vi "gui_T2.vi"(10 "input_xyz":T1) -> ()   [LabVIEW 2018]
uses:
  <vilib>/Analysis/NI_AALBase.lvlib
panel:
  in  "MW_power_db":dbl=1.0 caption="Width" min=0.0 max=10000.0 format="%#.3f"
  in  "MW_frequency_GHZ":dbl=1.0 caption="Width" min=0.0 max=10000.0 format="%#.3f"
  in  "Measurement_mode":enum16{"T2", "Rabi"}(ring)=enum."Rabi"
  in  "recenter_period_s":u32=5
  in  "recenter":bool=TRUE
  in  "show_all":bool
  in  "hide_all":bool
  out "elapsed_time_HMS":string
  in  "initial parameters":dbl[](array[numeric])=[0.5, 0.0001, 2.0, 100.0]
  out "estimated_time_HMS":string
  in  "plot_pulses":bool
  in  "gates_calculation":enum16{"Software", "Hardware"}(ring)=enum."Hardware"
  out "pulses":u32[][](graph)
  out "detections":u32[](graph)
  out "std. dev.":dbl format="%.3f"
  out "mean":dbl format="%0.2f"
  in  "auto_normalize":bool
  in  "normalize":bool
  in  "normalization_value":dbl=1.0 caption="Normalization value:" min=1.0 step=1.0
  out "status":string
  in  "use_proposed_width":bool
  in  "calc_width":bool
  in  "start":bool caption="Start"
  in  "save_file":bool
  out "contrast":dbl caption="Contrast :" format="%#_3f"
  in  "show_photons":bool
  in  "show_flags":bool
  out "mse":cluster{"read_widths_us":dbl[], "mse":dbl[]}(graph)
  in  "use_proposed_correction":bool
  out "proposed_read_width_us":dbl
  out "proposed_correction_us":dbl
  out "histogram":cluster{"histogram":i32[], "q_photons":i32[]}(graph)
  out "file_name":string caption="File name :"
  in  "sampling_mode":enum16{"Normal", "Sweep"}(ring)=enum."Sweep"
  out "quality":bool
  out "mse":dbl caption="Mean Square Error" format="%#.2e"
  out "T1_us":dbl format="%#.3g"
  out "T1 curves":cluster{dbl[], "dark_time_us":dbl[]}[](graph)
  in  "correction_us":dbl=0.65 caption="Delay"
  out "stop_count_photon":u32(colorbox)=16776704 caption="Stop Count & photon"
  out "stop_count":u32(colorbox)=6618880 caption="Stop Count"
  out "start_count_photon":u32(colorbox)=14417925 caption="Start Count & photon"
  out "start_count":u32(colorbox)=255 caption="Start Count"
  out "photon":u32(colorbox)=16448250 caption="Photon"
  out "noPhoton":u32(colorbox) caption="No Photon"
  out "photons_chart":u32[][](graph)
  in  "load_file":bool
  in  "refit":bool
  in  "read_width_us":dbl=1.0 caption="Width" min=0.0 max=10000.0 format="%#.3f"
  in  "read_delay_us":dbl caption="Delay"
  out "min_step":dbl format="%#.3f"
  in  "q_samples":i32=50
  in  "dt_stop_us":dbl=10000.0
  in  "dt_start_us":dbl=0.2
  in  "stop":bool
  in  "repetitions":i32=10000 caption="Repetitions" min=1 step=1
  in  "pulse_width_us":dbl=5.0 caption="Pulse width"
  # "Dark time [us]"
  # "*"
  # "*"
  # "us"
  # "*read_width_us and correction_us have to be multiple of 10ns\n*** start and stop markers are inside the detection gate. [start, stop]"
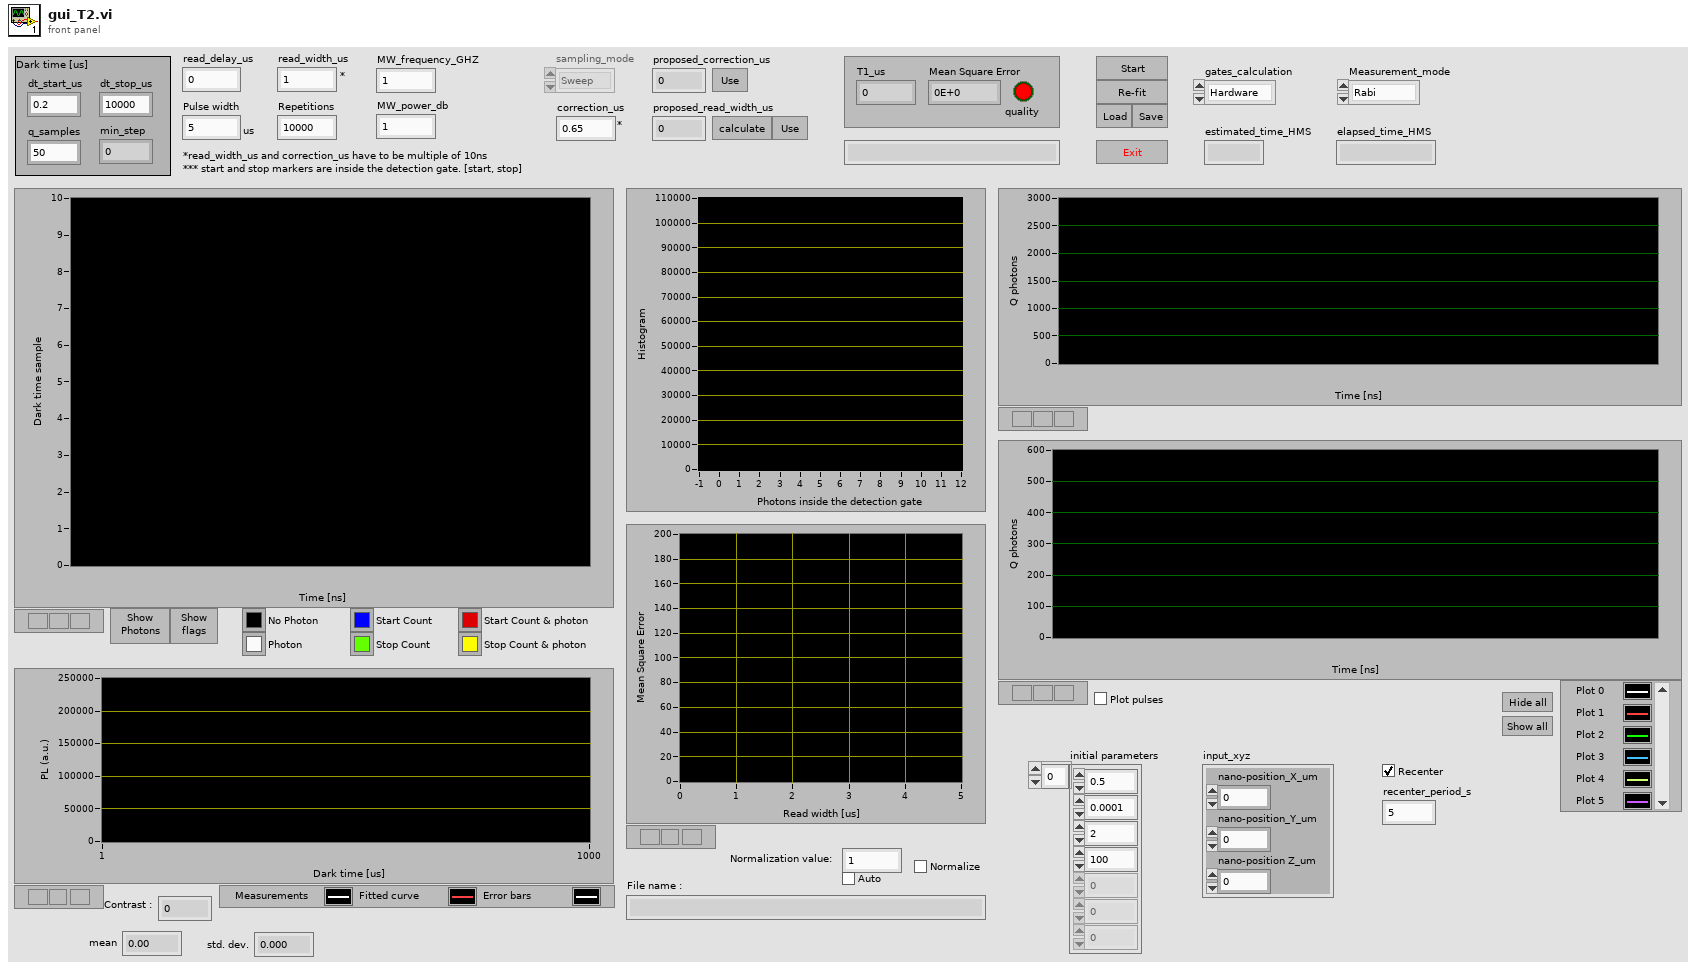
[diagram p1: front panel]
types:
  T1 = cluster{"nano-position_X_um":sgl, "nano-position_Y_um":sgl, "nano-position Z_um":sgl}
  T2 = cluster{"MW_power_db":dbl, "MW_frequency_GHZ":dbl}
  T3 = cluster{"MW_width_us":dbl[], "pulse_width_us":dbl, "read_delay_us":dbl, "read_width_us":dbl, "repetitions":i32, "sampling_mode":enum16{"Normal", "Sweep"}, "correction_us":dbl}
  T4 = cluster{"file_path":path, "file_name":string, "image":dbl[][][], "image_size_xy":cluster{"image_size_x_um":sgl, "image_size_y_um":sgl}, "pixel_dwell_time_ms":sgl, "Laser_power_mW":sgl, "pixel_size":dbl, "tile_ij":cluster{"tile_i":i32, "tile_j":i32}, "Objective":string, "ColorMarkers":cluster{dbl, u32}[], "timestamp":timestamp, "micro-position-xyz":cluster{"micro-position_x_mm":sgl, "micro-position_y_mm":sgl, "micro-position_z_mm":sgl}, "zero_xyz":cluster{"zero_x_mm":dbl, "zero_y_mm":dbl, "zero_z_mm":dbl}, "nano-position-xyz":cluster{"nano-position_x_V":sgl, "nano-position_y_V":sgl, "nano-position_z_V":sgl}, "Kxyz":cluster{"Kx_V/um":sgl, "Ky_V/um":sgl, "Kz_V/um":sgl}}
  T5 = cluster{"x_um":sgl[], "y_um":sgl[], "z_um":sgl[], "timetag":timestamp[]}
  T6 = cluster{"sampling_times":dbl[], "fitted_signal":dbl[]}
  T7 = cluster{"Ie":dbl, "Cm":dbl, "Tm":dbl, "C1":dbl, "T1":dbl, "mse":dbl}
  T8 = cluster{"dark_times_us":dbl[], "pulse_width_us":dbl, "read_delay_us":dbl, "read_width_us":dbl, "repetitions":i32, "sampling_mode":enum16{"Normal", "Sweep"}, "correction_us":dbl}
  T9 = cluster{"input_xyz":cluster{"nano-position_X_um":sgl, "nano-position_Y_um":sgl, "nano-position Z_um":sgl}, "recenter":bool, "recenter_s":u32}
  T10 = enum16{"standby", "doT1", "abort", "save", "re-fit", "load", "refresh", "use_proposed", "calcWidth"}
  T11 = cluster{"dark_times":dbl[], "fitted_signal":dbl[]}
  T12 = cluster{"dark_times_us":dbl[], "measured_signal":dbl[]}
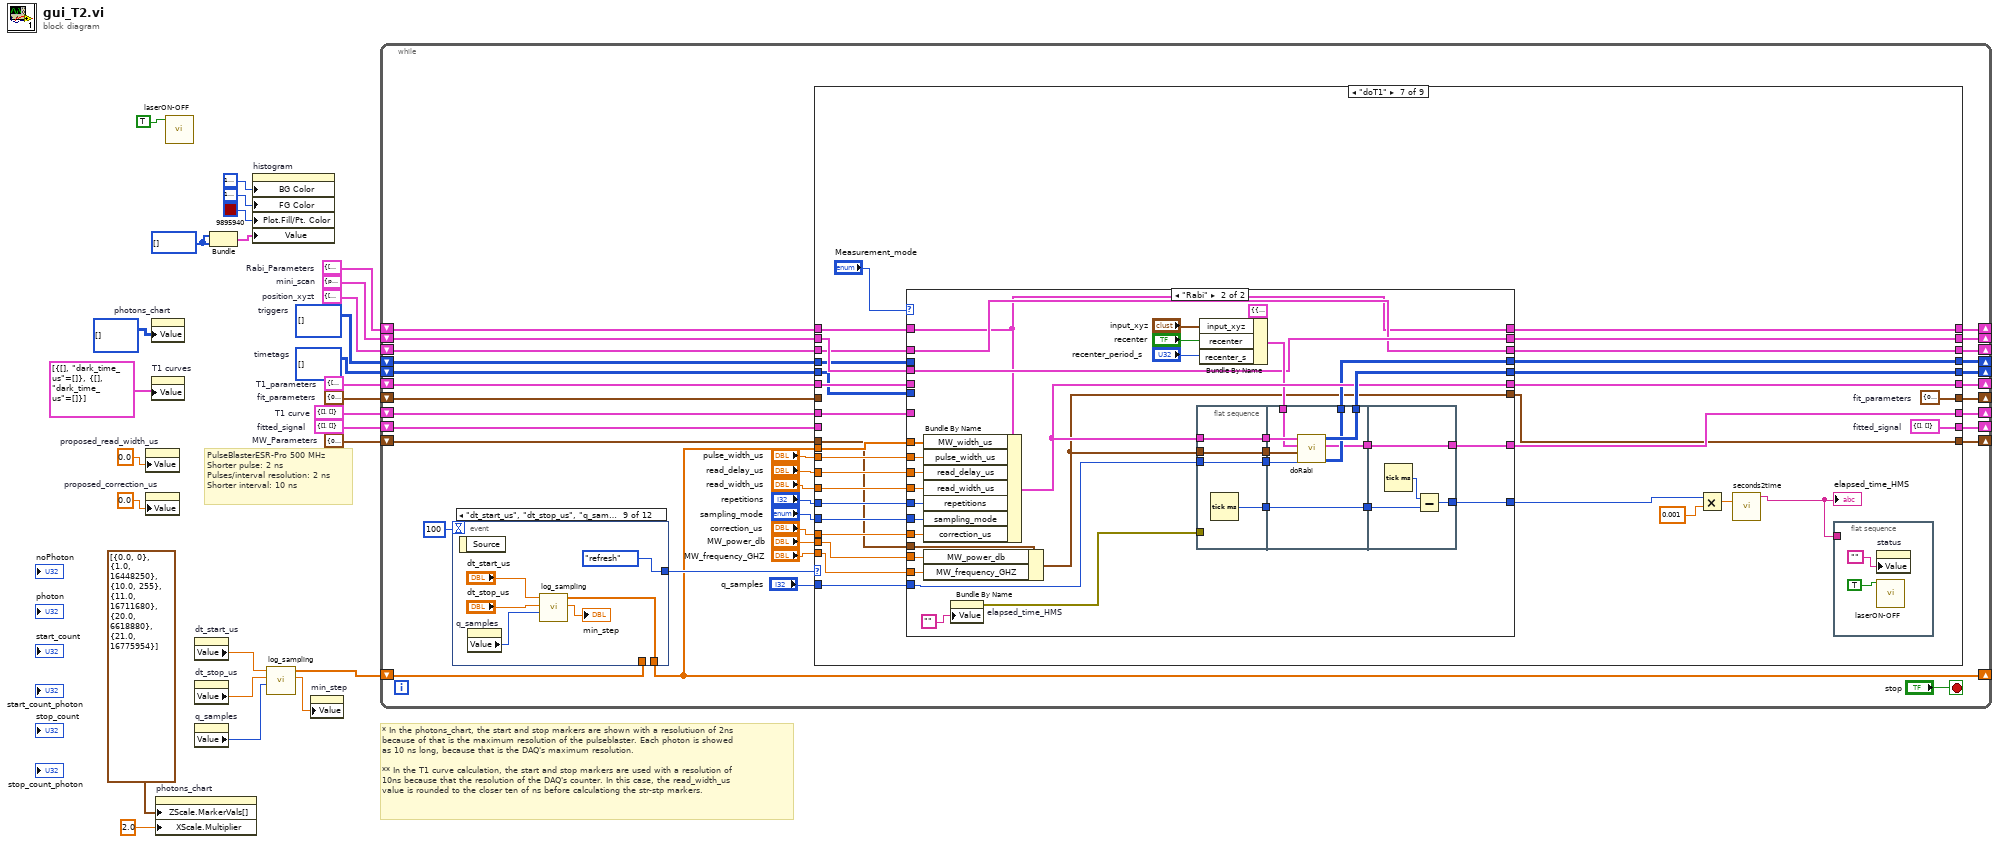
[diagram p0: block diagram]
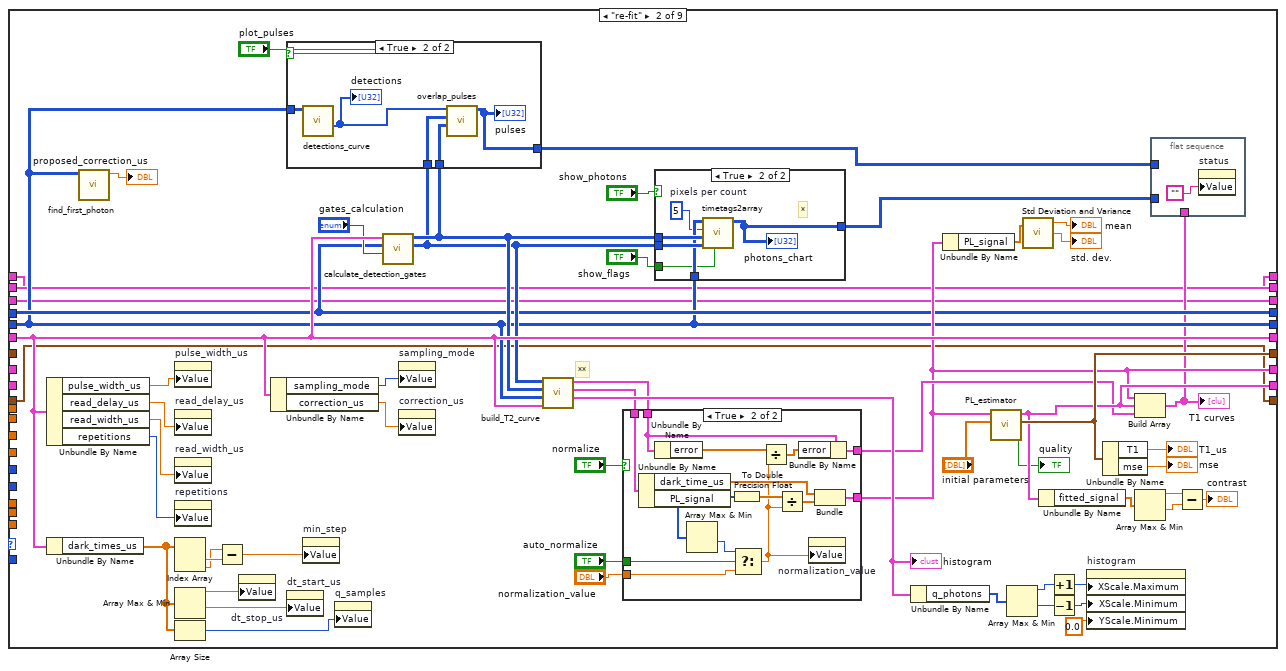
[diagram p3: hidden frame]
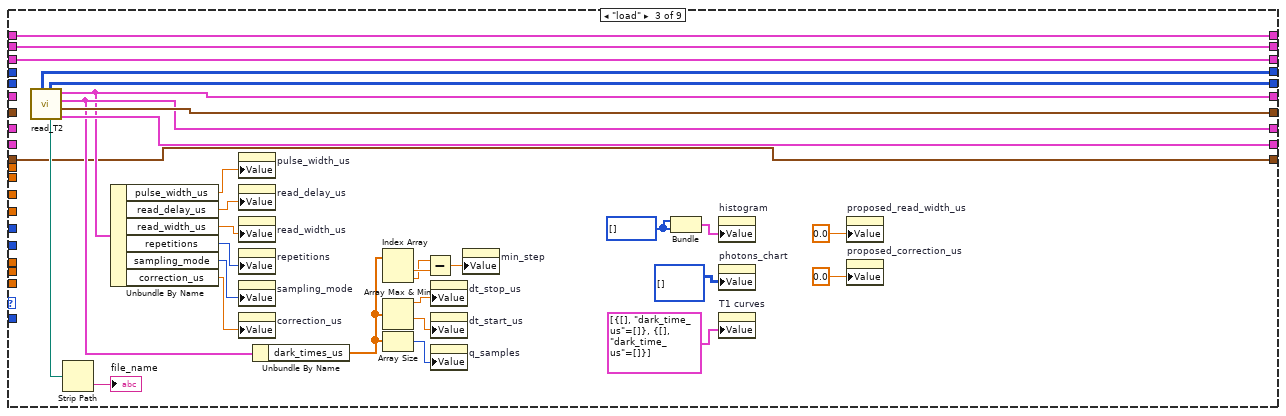
[diagram p7: hidden frame]
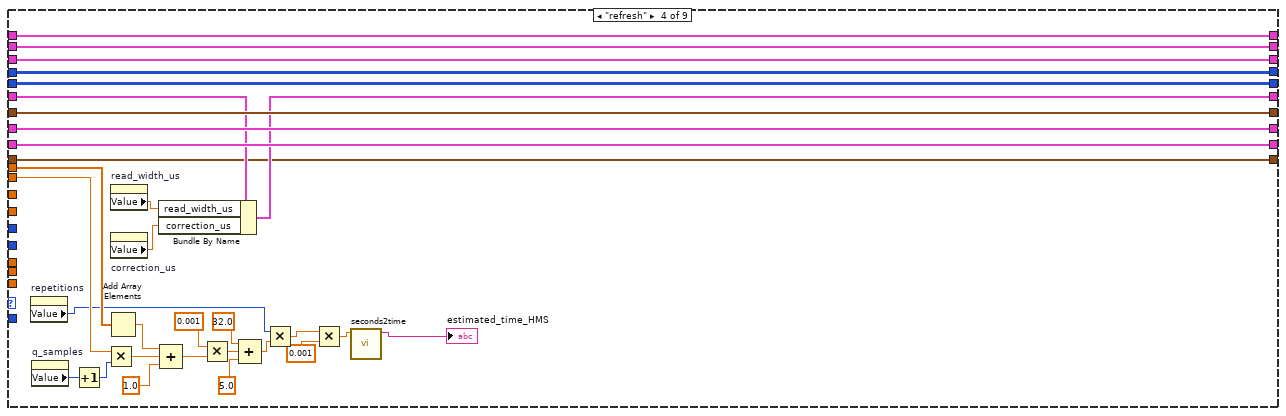
[diagram p8: hidden frame]
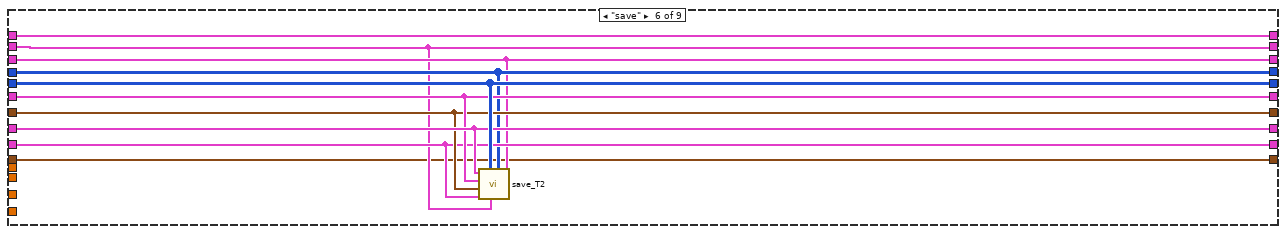
[diagram p10: hidden frame]
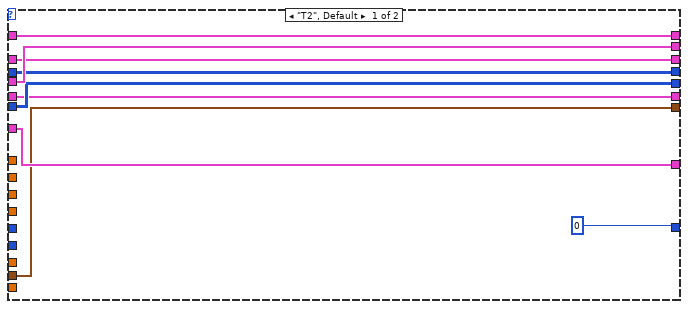
[diagram p11: hidden frame]
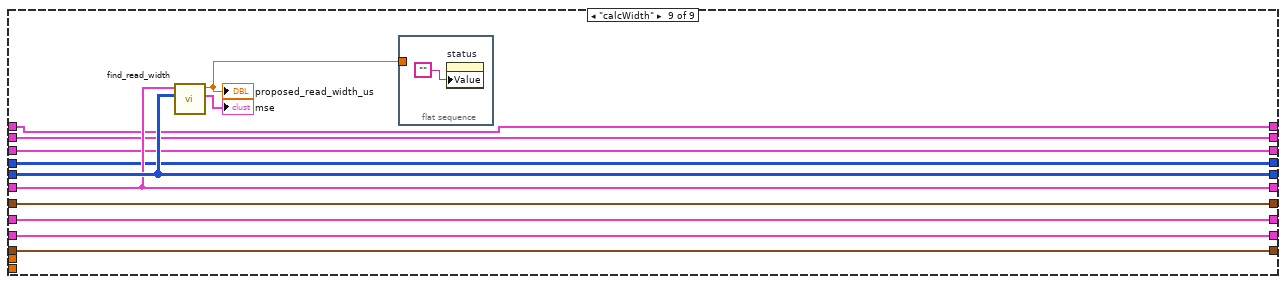
[diagram p13: hidden frame]
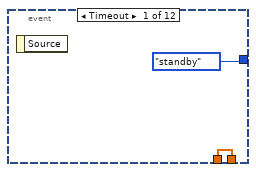
[diagram p14: hidden frame]
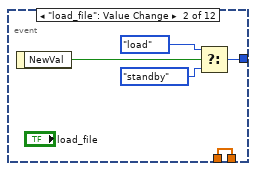
[diagram p15: hidden frame]
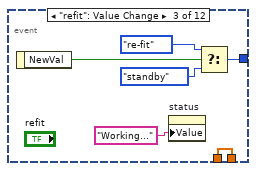
[diagram p16: hidden frame]
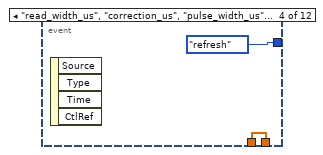
[diagram p17: hidden frame]
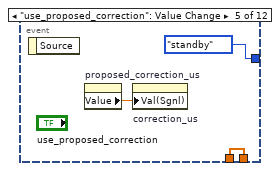
[diagram p18: hidden frame]
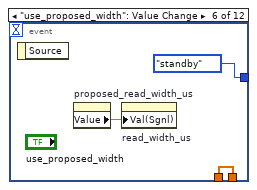
[diagram p19: hidden frame]
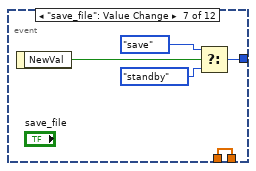
[diagram p20: hidden frame]
diagram:
  w1 = T2 {"MW_power_db"=0.0, "MW_frequency_GHZ"=0.0}  # MW_Parameters
  w2 = T3 {"MW_width_us"=[], "pulse_width_us"=0.0, "read_delay_us"=0.0, "read_width_us"=0.0, "repetitions"=0, "sampling_mode"=enum."Normal", "correction_us"=0.0}  # Rabi_Parameters
  w3 = T4 {"file_path"=path "", "file_name"="", "image"=[], "image_size_xy"={"image_size_x_um"=0.0, "image_size_y_um"=0.0}, "pixel_dwell_time_ms"=0.0, "Laser_power_mW"=0.0, "pixel_size"=0.0, "tile_ij"={"tile_i"=0, "tile_j"=0}, "Objective"="", "ColorMarkers"=[], "timestamp"=timestamp(0 s since 1904-01-01), "micro-position-xyz"={"micro-position_x_mm"=0.0, "micro-position_y_mm"=0.0, "micro-position_z_mm"=0.0}, "zero_xyz"={"zero_x_mm"=0.0, "zero_y_mm"=0.0, "zero_z_mm"=0.0}, "nano-position-xyz"={"nano-position_x_V"=0.0, "nano-position_y_V"=0.0, "nano-position_z_V"=0.0}, "Kxyz"={"Kx_V/um"=0.0, "Ky_V/um"=0.0, "Kz_V/um"=0.0}}  # mini_scan
  w4 = T5 {"x_um"=[], "y_um"=[], "z_um"=[], "timetag"=[]}  # position_xyzt
  w6 = u32[][] []  # triggers
  w24 = T6 {"sampling_times"=[], "fitted_signal"=[]}  # fitted_signal
  w7 = u32[][] []  # timetags
  w25 = cluster{dbl[], "dark_time_us":dbl[]} {[], "dark_time_us"=[]}  # T1 curve
  w26 = T7 {"Ie"=0.0, "Cm"=0.0, "Tm"=0.0, "C1"=0.0, "T1"=0.0, "mse"=0.0}  # fit_parameters
  w23 = T8 {"dark_times_us"=[], "pulse_width_us"=0.0, "read_delay_us"=0.0, "read_width_us"=0.0, "repetitions"=0, "sampling_mode"=enum."Normal", "correction_us"=0.0}  # T1_parameters
  w18 = i32[] []
  # "* In the photons_chart, the start and stop markers are shown with a resolutiuon of 2ns \nbecause of that is the maximum resolution of the pulseblaster. Each photon is showed\nas 10 ns long, because that is the DAQ's maximum resolution.\n\n** In the T1 curve calculation, the start and stop markers are used with a resolution of\n10ns because that the resolution of the DAQ's counter. In this case, the read_width_us\nvalue is rounded to the closer ten of ns before calculationg the str-stp markers."
  # "PulseBlasterESR-Pro 500 MHz \nShorter pulse: 2 ns\nPulses/interval resolution: 2 ns\nShorter interval: 10 ns"
  n1 = property on="proposed_read_width_us" class="DigNum (strict)"("Value"=0.0 ("proposed_read_width_us")) -> ()  [unwired: 2 in, 2 out]
  n2 = property on="proposed_correction_us" class="DigNum (strict)"("Value"=0.0 ("proposed_correction_us")) -> ()  [unwired: 2 in, 2 out]
  n3 = property on="photons_chart" class="IntGraph (strict)"("Value"=i32[][] []) -> ()  [unwired: 2 in, 2 out]
  n4 = property on="T1 curves" class="XYGraph (strict)"("Value"=cluster{dbl[], "dark_time_us":dbl[]}[] [{[], "dark_time_us"=[]}, {[], "dark_time_us"=[]}] ("T1 curves")) -> ()  [unwired: 2 in, 2 out]
  n5 = property on="photons_chart" class="IntGraph (strict)"("ZScale.MarkerVals[]"=cluster{dbl, u32}[] [{0.0, 0}, {1.0, 16448250}, {10.0, 255}, {11.0, 16711680}, {20.0, 6618880}, {21.0, 16775954}] ("Z Scale.Marker Values[]"), "XScale.Multiplier"=2.0 ("X Scale.Offset and Multiplier:Multiplier")) -> ()  [unwired: 2 in, 2 out]
  n6 = call "laserON-OFF.vi"("ON-OFF"=TRUE) -> ()  [unwired: 11 in]
  n7 = property on="dt_start_us" class="DigNum (strict)"() -> ("Value"=w10:dbl)  [unwired: 2 in, 2 out]
  n8 = property on="dt_stop_us" class="DigNum (strict)"() -> ("Value"=w11:dbl)  [unwired: 2 in, 2 out]
  n9 = property on="q_samples" class="DigNum (strict)"() -> ("Value"=w12:i32)  [unwired: 2 in, 2 out]
  n10 = Bundle(w18, w18) -> (w17:cluster{i32[], i32[]})  [unwired: 1 in]
  n11 = property on="histogram" class="XYGraph (strict)"("BG Color"=u32 16777222 ("Plot Area:Colors:FG Color"), "FG Color"=u32 16777228 ("Plot Area:Colors:FG Color"), "Plot.Fill/Pt. Color"=u32 9895940 ("Plot Area:Colors:FG Color"), "Value"=w17) -> ()  [unwired: 2 in, 2 out]
  n12 = call "log_sampling.vi"("q_samples"=w12, "stop_us"=w11, "start_us"=w10) -> ("min_step_us"=w13:dbl, "sampling_times_us"=w9:dbl[])  [unwired: 7 in]
  n13 = property on="min_step" class="DigNum (strict)"("Value"=w13) -> ()  [unwired: 2 in, 2 out]
  n14 = while {
    shift-right: [w51] -> _
    shift-left: w23 -> [w58]
    shift-right: [w50] -> _
    shift-left: w26 -> [w57]
    shift-right: [w49] -> _
    shift-left: w25 -> [w56]
    shift-right: [w55] -> _
    shift-left: w24 -> [w54]
    shift-right: [w52] -> _
    shift-left: w7 -> [w53]
    shift-right: [w41] -> _
    shift-left: w9 -> [w42]
    shift-right: [w40] -> _
    shift-left: w6 -> [w39]
    shift-right: [w38] -> _
    shift-left: w4 -> [w37]
    shift-right: [w35] -> _
    shift-left: w3 -> [w36]
    shift-right: [w33] -> _
    shift-left: w2 -> [w34]
    shift-right: [w29] -> _
    shift-left: w1 -> [w32]
    stop <- "stop" stop-if-true
    n15 = event shown="[8] \"dt_start_us\", \"dt_stop_us\", \"q_samples\": Value Change" {
      selector: _ -> [_ _ _ _ _ _ _ _ _ _ _ _]
      dyn-events: _ -> [_ _ _ _ _ _ _ _ _ _ _ _]
      timeout: 100 -> [_ _ _ _ _ _ _ _ _ _ _ _]
      tunnel: [T10."standby" w360 w366 T10."refresh" T10."standby" T10."standby" w379 w386 T10."refresh" w398 T10."standby" T10."standby"] -> w59
      tunnel: w42 -> [w355 w357 w363 w368 w370 w373 w376 w381 _ w394 w401 w407]
      tunnel: [w355 w357 w363 w368 w370 w373 w376 w381 w388 w394 w401 w407] -> w41
      event Timeout {
        n16 = event-data() -> ()  [unwired: 1 in, 1 out]
      }
      event "load_file": Value Change {
        n17 = event-data() -> ("NewVal"=w361:bool)  [unwired: 1 in]
        n18 = Select(t=T10."load", s=w361, f=T10."standby") -> (s? t:f=w360:T10)
      }
      event "refit": Value Change {
        n19 = event-data() -> ("NewVal"=w367:bool)  [unwired: 1 in]
        n20 = property on="status" class="Str"("Value"="Working...") -> ()  [unwired: 2 in, 2 out]
        n21 = Select(t=T10."re-fit", s=w367, f=T10."standby") -> (s? t:f=w366:T10)
      }
      event "read_width_us", "correction_us", "pulse_width_us", "repetitions": Value Change {
        n22 = event-data() -> ()  [unwired: 1 in, 4 out]
      }
      event "use_proposed_correction": Value Change {
        n23 = event-data() -> ()  [unwired: 1 in, 1 out]
        n24 = property on="proposed_correction_us" class="DigNum (strict)"() -> ("Value"=w372:dbl)  [unwired: 2 in, 2 out]
        n25 = property on="correction_us" class="DigNum (strict)"("Val(Sgnl)"=w372) -> ()  [unwired: 2 in, 2 out]
      }
      event "use_proposed_width": Value Change {
        n26 = event-data() -> ()  [unwired: 1 in, 1 out]
        n27 = property on="proposed_read_width_us" class="DigNum (strict)"() -> ("Value"=w375:dbl)  [unwired: 2 in, 2 out]
        n28 = property on="read_width_us" class="DigNum (strict)"("Val(Sgnl)"=w375) -> ()  [unwired: 2 in, 2 out]
      }
      event "save_file": Value Change {
        n29 = event-data() -> ("NewVal"=w380:bool)  [unwired: 1 in]
        n30 = Select(t=T10."save", s=w380, f=T10."standby") -> (s? t:f=w379:T10)
      }
      event "start": Value Change {
        n31 = event-data() -> ("NewVal"=w385:bool)  [unwired: 1 in]
        n32 = Select(t=T10."doT1", s=w385, f=T10."standby") -> (s? t:f=w386:T10)
        "status" <- "Working..."
      }
      event "dt_start_us", "dt_stop_us", "q_samples": Value Change {
        n33 = event-data() -> ()  [unwired: 1 in, 1 out]
        n34 = property on="q_samples" class="DigNum (strict)"() -> ("Value"=w387:i32)  [unwired: 2 in, 2 out]
        n35 = call "log_sampling.vi"("q_samples"=w387, "stop_us"="dt_stop_us", "start_us"="dt_start_us") -> ("min_step_us"=→"min_step":dbl, "sampling_times_us"=w388:dbl[])  [unwired: 7 in]
      }
      event "calc_width": Value Change {
        n36 = event-data() -> ("NewVal"=w397:bool)  [unwired: 1 in]
        n37 = property on="status" class="Str"("Value"="Working...") -> ()  [unwired: 2 in, 2 out]
        n38 = Select(t=T10."calcWidth", s=w397, f=T10."standby") -> (s? t:f=w398:T10)
      }
      event "hide_all": Value Change {
        n39 = event-data() -> ()  [unwired: 1 in, 1 out]
        n40 = property on="q_samples" class="DigNum (strict)"() -> ("Value"=w399:i32)  [unwired: 2 in, 2 out]
        n41 = Increment(x=w399) -> (x+1=w400:i32)
        n42 = for {
          N: w400 -> [_]
          i -> [w404]
          n43 = property on="pulses" class="WFGraph (strict)"("Active Plot"=w404, "Plot.Visible?"=FALSE ("Plot.Visible")) -> ()  [unwired: 2 in, 2 out]
        }
      }
      event "show_all": Value Change {
        n44 = event-data() -> ()  [unwired: 1 in, 1 out]
        n45 = property on="q_samples" class="DigNum (strict)"() -> ("Value"=w405:i32)  [unwired: 2 in, 2 out]
        n46 = Increment(x=w405) -> (x+1=w406:i32)
        n47 = for {
          N: w406 -> [_]
          i -> [w410]
          n48 = property on="pulses" class="WFGraph (strict)"("Active Plot"=w410, "Plot.Visible?"=TRUE ("Plot.Visible")) -> ()  [unwired: 2 in, 2 out]
        }
      }
    }
    n49 = case shown="\"doT1\"" w59 {
      tunnel: w58 -> [w71 w105 _ w214 w227 w236 w271 w340 w351]
      tunnel: w57 -> [w70 _ _ w217 w226 w235 _ w339 w350]
      tunnel: w56 -> [w69 _ _ w216 w225 w237 w245 w338 w349]
      tunnel: [w68 w102 w187 w215 w224 w234 w257 w337 w348] -> w55
      tunnel: w54 -> [w68 _ _ w215 w224 w234 _ w337 w348]
      tunnel: [w67 w79 w178 w218 w228 w238 w270 w341 w352] -> w52
      tunnel: w53 -> [w67 w79 _ w218 w228 w238 w246 w341 w352]
      tunnel: [w71 w105 w180 w213 w227 w236 w261 w340 w351] -> w51
      tunnel: [w70 w128 w186 w217 w226 w235 w256 w339 w350] -> w50
      tunnel: [w69 w89 w185 w216 w225 w237 w262 w338 w349] -> w49
      tunnel: "read_delay_us" -> [_ _ _ _ _ _ w269 _ _]
      tunnel: "pulse_width_us" -> [_ _ _ w208 _ _ w268 _ _]
      tunnel: "read_width_us" -> [_ _ _ _ _ _ w267 _ _]
      tunnel: "repetitions" -> [_ _ _ _ _ _ w266 _ _]
      tunnel: "sampling_mode" -> [_ _ _ _ _ _ w265 _ _]
      tunnel: "correction_us" -> [_ _ _ _ _ _ w264 _ _]
      tunnel: w41 -> [_ _ _ w209 _ _ w263 _ _]
      tunnel: [w66 w80 w161 w210 w223 w233 w260 w336 w346] -> w40
      tunnel: w39 -> [w66 w80 _ w210 w223 w233 w247 w336 w346]
      tunnel: [w65 w75 w160 w191 w222 w232 w253 w335 w345] -> w38
      tunnel: w37 -> [w65 w75 w160 w191 w222 w232 w248 w335 w345]
      tunnel: [w64 w74 w159 w190 w221 w231 w252 w334 w344] -> w35
      tunnel: w36 -> [w64 w74 w159 w190 w221 w231 w249 w334 w344]
      tunnel: w34 -> [w63 w73 w158 w189 w220 w230 w250 w333 w343]
      tunnel: [w63 w73 w158 w189 w220 w230 w244 w333 w343] -> w33
      tunnel: w32 -> [w62 w72 w157 w188 w219 w229 w243 w332 w342]
      tunnel: "MW_power_db" -> [_ _ _ _ _ _ w242 _ _]
      tunnel: "MW_frequency_GHZ" -> [_ _ _ _ _ _ w241 _ _]
      tunnel: [w62 w72 w157 w188 w219 w229 w240 w332 w342] -> w29
      tunnel: "q_samples" -> [_ _ _ _ _ _ w239 _ _]
      frame "standby", Default {
      }
      frame "re-fit" {
        # "**"
        n50 = Unbundle By Name(w105) -> ("pulse_width_us"=w120:dbl, "read_delay_us"=w119:dbl, "read_width_us"=w118:dbl, "repetitions"=w117:i32)
        n51 = Unbundle By Name(w105) -> ("dark_times_us"=w125:dbl[])
        n52 = call "find_first_photon.vi"("timetags"=w79) -> ("Numeric"=→"proposed_correction_us":dbl)  [unwired: 10 in]
        n53 = property on="pulse_width_us" class="DigNum (strict)"("Value"=w120) -> ()  [unwired: 2 in, 2 out]
        n54 = property on="read_delay_us" class="DigNum (strict)"("Value"=w119) -> ()  [unwired: 2 in, 2 out]
        n55 = property on="read_width_us" class="DigNum (strict)"("Value"=w118) -> ()  [unwired: 2 in, 2 out]
        n56 = property on="repetitions" class="DigNum (strict)"("Value"=w117) -> ()  [unwired: 2 in, 2 out]
        n57 = Index Array(array=w125) -> (element #1=w127:dbl, element #2=w126:dbl)  [unwired: 2 in]
        n58 = Array Max & Min(array=w125) -> (max value=w124:dbl, min value=w123:dbl)  [unwired: 2 out]
        n59 = Array Size(array=w125) -> (size(s)=w122:i32)
        n60 = Subtract(x=w126, y=w127) -> (x-y=w121:dbl)
        n61 = property on="dt_stop_us" class="DigNum (strict)"("Value"=w124) -> ()  [unwired: 2 in, 2 out]
        n62 = Unbundle By Name(w105) -> ("sampling_mode"=w115:enum16{"Normal", "Sweep"}, "correction_us"=w114:dbl)
        n63 = property on="dt_start_us" class="DigNum (strict)"("Value"=w123) -> ()  [unwired: 2 in, 2 out]
        n64 = property on="min_step" class="DigNum (strict)"("Value"=w121) -> ()  [unwired: 2 in, 2 out]
        n65 = property on="q_samples" class="DigNum (strict)"("Value"=w122) -> ()  [unwired: 2 in, 2 out]
        n66 = call "calculate_detection_gates.vi"("gates_calculation"="gates_calculation", "triggers"=w80, "T1_parameters"=w105) -> ("start_read"=w84:u32[][], "stop_read"=w85:u32[][])  [unwired: 7 in]
        n67 = case shown="True" "plot_pulses" {
          tunnel: w85 -> [_ w134]
          tunnel: w84 -> [_ w133]
          tunnel: w79 -> [_ w132]
          tunnel: [_ w130] -> w76
          frame False {
          }
          frame True {
            n68 = call "detections_curve.vi"("timetags"=w132) -> ("detections"=w131:u32[])  [unwired: 10 in]
            "detections" <- w131
            n69 = call "overlap_pulses.vi"("stop_read"=w134, "start_read"=w133, "detections"=w131) -> ("pulses"=w130:u32[][])  [unwired: 8 in]
            "pulses" <- w130
          }
        }
        n70 = property on="sampling_mode" class="Enum (strict)"("Value"=w115) -> ()  [unwired: 2 in, 2 out]
        n71 = property on="correction_us" class="DigNum (strict)"("Value"=w114) -> ()  [unwired: 2 in, 2 out]
        n72 = call "build_T2_curve.vi"("T1_parameters"=w105, "timetags"=w79, "stop_read"=w85, "start_read"=w84) -> ("histogram"=w113:cluster{"q_photons":i32[], "histogram":i32[]}, "T1 curve"=w83:cluster{"dark_time_us":dbl[], "PL_signal":i32[]}, "error_bars"=w92:cluster{"dark_times_us":dbl[], "error":dbl[]})  [unwired: 5 in]
        "histogram" <- w113
        n73 = case shown="True" "normalize" {
          tunnel: [w135 w150] -> w89
          tunnel: "normalization_value" -> [_ w141]
          tunnel: w92 -> [w136 w145]
          tunnel: [w136 w143] -> w91
          tunnel: "auto_normalize" -> [_ w139]
          tunnel: w83 -> [w135 w137]
          frame False {
          }
          frame True {
            n74 = Unbundle By Name(w137) -> ("dark_time_us"=w148:dbl[], "PL_signal"=w142:i32[])
            n75 = Unbundle By Name(w145) -> ("error"=w146:dbl[])
            n76 = Array Max & Min(array=w142) -> (min value=w140:i32)  [unwired: 3 out]
            n77 = To Double Precision Float(number=w142) -> (double precision float=w147:dbl[])
            n78 = Select(t=w140, s=w139, f=w141) -> (s? t:f=w138:dbl)
            n79 = Divide(x=w146, y=w138) -> (x/y=w144:dbl[])
            n80 = Divide(x=w147, y=w138) -> (x/y=w149:dbl[])
            n81 = Bundle By Name(cluster=w145, "error"=w144) -> (w143:cluster{"dark_times_us":dbl[], "error":dbl[]})
            n82 = property on="normalization_value" class="DigNum (strict)"("Value"=w138) -> ()  [unwired: 2 in, 2 out]
            n83 = Bundle("dark_time_us"=w148, w149) -> (w150:cluster{"dark_time_us":dbl[], dbl[]})  [unwired: 1 in]
          }
        }
        n84 = case shown="True" "show_photons" {
          tunnel: w84 -> [_ w156]
          tunnel: w85 -> [_ w155]
          tunnel: w79 -> [_ w154]
          tunnel: "show_flags" -> [_ w153]
          tunnel: [_ w151] -> w77
          frame False {
          }
          frame True {
            w152 = u32 5  # pixels per count
            # "*"
            n85 = call "timetags2array.vi"("show_flags"=w153, "start_read"=w156, "stop_read"=w155, "pixels/count"=w152, "timetags"=w154) -> ("photons_chart"=w151:u32[][])  [unwired: 6 in]
            "photons_chart" <- w151
          }
        }
        n86 = Unbundle By Name(w113) -> ("q_photons"=w112:i32[])
        n87 = Unbundle By Name(w89) -> ("PL_signal"=w88:dbl[])
        n88 = call "PL_estimator.vi"("initial parameters"="initial parameters", "measured_signal"=w89) -> ("quality_check"=→"quality":bool, "fit_parameters"=w128:T7, "fitted_signal"=w102:T6)  [unwired: 7 in]
        n89 = Array Max & Min(array=w112) -> (max value=w111:i32, min value=w109:i32)  [unwired: 2 out]
        n90 = call <vilib>:"Std Deviation and Variance.vi"("X"=w88) -> ("mean"=→"mean":dbl, "standard deviation"=→"std. dev.":dbl)  [unwired: 1 in, 1 out]
        n91 = Unbundle By Name(w102) -> ("fitted_signal"=w101:dbl[])
        n92 = Increment(x=w111) -> (x+1=w110:i32)
        n93 = Decrement(x=w109) -> (x-1=w108:i32)
        n94 = property on="histogram" class="XYGraph (strict)"("XScale.Maximum"=w110, "XScale.Minimum"=w108, "YScale.Minimum"=0.0 ("Y Scale.Range:Minimum")) -> ()  [unwired: 2 in, 2 out]
        n95 = Unbundle By Name(w128) -> ("T1"=→"T1_us":dbl, "mse"=→"mse":dbl)
        n96 = Build Array(w89, w102, w91) -> (w78:cluster{"dark_times_us":dbl[], "error":dbl[]}[])
        "T1 curves" <- w78
        n97 = Array Max & Min(array=w101) -> (max value=w100:dbl, min value=w99:dbl)  [unwired: 2 out]
        n98 = flat-sequence {
          tunnel: w78 -> [_]
          tunnel: w77 -> [_]
          tunnel: w76 -> [_]
          frame #0 {
            n99 = property on="status" class="Str"("Value"="") -> ()  [unwired: 2 in, 2 out]
          }
        }
        n100 = Subtract(x=w100, y=w99) -> (x-y=→"contrast":dbl)
      }
      frame "load" {
        w175 = i32[] []
        n101 = call "read_T2.vi"() -> ("fitted_signal"=w187:T11, "fit_parameters"=w186:T7, "T1_curve"=w185:T12, "T1_parameters"=w180:T8, "file_path"=w177:path, "timetags"=w178:u32[][], "triggers"=w161:u32[][])  [unwired: 5 in]
        n102 = Strip Path(path=w177) -> (name=→"file_name":string)  [unwired: 1 out]
        n103 = Unbundle By Name(w180) -> ("pulse_width_us"=w169:dbl, "read_delay_us"=w168:dbl, "read_width_us"=w181:dbl, "repetitions"=w166:i32, "sampling_mode"=w167:enum16{"Normal", "Sweep"}, "correction_us"=w179:dbl)
        n104 = property on="pulse_width_us" class="DigNum (strict)"("Value"=w169) -> ()  [unwired: 2 in, 2 out]
        n105 = property on="read_delay_us" class="DigNum (strict)"("Value"=w168) -> ()  [unwired: 2 in, 2 out]
        n106 = property on="read_width_us" class="DigNum (strict)"("Value"=w181) -> ()  [unwired: 2 in, 2 out]
        n107 = property on="repetitions" class="DigNum (strict)"("Value"=w166) -> ()  [unwired: 2 in, 2 out]
        n108 = property on="sampling_mode" class="Enum (strict)"("Value"=w167) -> ()  [unwired: 2 in, 2 out]
        n109 = property on="correction_us" class="DigNum (strict)"("Value"=w179) -> ()  [unwired: 2 in, 2 out]
        n110 = Unbundle By Name(w185) -> ("dark_times_us"=w184:dbl[])
        n111 = Index Array(array=w184) -> (element #1=w183:dbl, element #2=w182:dbl)  [unwired: 2 in]
        n112 = Array Max & Min(array=w184) -> (max value=w163:dbl, min value=w164:dbl)  [unwired: 2 out]
        n113 = Array Size(array=w184) -> (size(s)=w165:i32)
        n114 = Subtract(x=w182, y=w183) -> (x-y=w162:dbl)
        n115 = property on="dt_stop_us" class="DigNum (strict)"("Value"=w163) -> ()  [unwired: 2 in, 2 out]
        n116 = property on="dt_start_us" class="DigNum (strict)"("Value"=w164) -> ()  [unwired: 2 in, 2 out]
        n117 = property on="q_samples" class="DigNum (strict)"("Value"=w165) -> ()  [unwired: 2 in, 2 out]
        n118 = property on="min_step" class="DigNum (strict)"("Value"=w162) -> ()  [unwired: 2 in, 2 out]
        n119 = Bundle(w175, w175) -> (w174:cluster{i32[], i32[]})  [unwired: 1 in]
        n120 = property on="histogram" class="XYGraph (strict)"("Value"=w174) -> ()  [unwired: 2 in, 2 out]
        n121 = property on="photons_chart" class="IntGraph (strict)"("Value"=i32[][] []) -> ()  [unwired: 2 in, 2 out]
        n122 = property on="T1 curves" class="XYGraph (strict)"("Value"=cluster{dbl[], "dark_time_us":dbl[]}[] [{[], "dark_time_us"=[]}, {[], "dark_time_us"=[]}] ("T1 curves")) -> ()  [unwired: 2 in, 2 out]
        n123 = property on="proposed_read_width_us" class="DigNum (strict)"("Value"=0.0 ("proposed_read_width_us")) -> ()  [unwired: 2 in, 2 out]
        n124 = property on="proposed_correction_us" class="DigNum (strict)"("Value"=0.0 ("proposed_correction_us")) -> ()  [unwired: 2 in, 2 out]
      }
      frame "refresh" {
        n125 = property on="repetitions" class="DigNum (strict)"() -> ("Value"=w196:i32)  [unwired: 2 in, 2 out]
        n126 = property on="q_samples" class="DigNum (strict)"() -> ("Value"=w207:i32)  [unwired: 2 in, 2 out]
        n127 = Increment(x=w207) -> (x+1=w206:i32)
        n128 = Multiply(x=w208, y=w206) -> (x*y=w204:dbl)
        n129 = Add Array Elements(numeric array=w209) -> (sum=w205:dbl)
        n130 = property on="read_width_us" class="DigNum (strict)"() -> ("Value"=w212:dbl)  [unwired: 2 in, 2 out]
        n131 = property on="correction_us" class="DigNum (strict)"() -> ("Value"=w211:dbl)  [unwired: 2 in, 2 out]
        n132 = Bundle By Name(cluster=w214, "read_width_us"=w212, "correction_us"=w211) -> (w213:T8)
        n133 = Compound Arithmetic op=ADD(w205, w204, 1.0 ("value")) -> (w202:dbl)
        n134 = Multiply(x=0.001, y=w202) -> (x*y=w200:dbl)
        n135 = Compound Arithmetic op=ADD(32.0 ("value"), w200, 5.0 ("value")) -> (w197:dbl)
        n136 = Multiply(x=w196, y=w197) -> (x*y=w195:dbl)
        n137 = Multiply(x=w195, y=0.001 ("x")) -> (x*y=w193:dbl)
        n138 = call "seconds2time.vi"("seconds"=w193) -> ("HH:MM:SS"=→"estimated_time_HMS":string)  [unwired: 10 in]
      }
      frame "use_proposed" {
      }
      frame "save" {
        n139 = call "save_T2.vi"("position_xyzt"=w232, "triggers"=w233, "image_info"=w231, "timetags"=w238, "fitted_signal_in"=w234, "fit_parameters"=w235, "T1_parameters"=w236, "T1_curve_in"=w237) -> ()  [unwired: 4 in]
      }
      frame "doT1" {
        w256 = T7 {"Ie"=0.0, "Cm"=0.0, "Tm"=0.0, "C1"=0.0, "T1"=0.0, "mse"=0.0}  # fit_parameters
        w257 = T6 {"sampling_times"=[], "fitted_signal"=[]}  # fitted_signal
        n140 = case shown="\"Rabi\"" "Measurement_mode" {
          tunnel: w271 -> [w276 _]
          tunnel: [w277 w309] -> w270
          tunnel: w269 -> [_ w308]
          tunnel: w268 -> [_ w307]
          tunnel: w267 -> [_ w306]
          tunnel: w266 -> [_ w305]
          tunnel: w265 -> [_ w304]
          tunnel: w264 -> [_ w303]
          tunnel: w263 -> [_ w302]
          tunnel: [w275 w301] -> w262
          tunnel: [w276 w300] -> w261
          tunnel: [w278 w299] -> w260
          tunnel: [0 w296] -> w254
          tunnel: [w279 w289] -> w253
          tunnel: [w280 w290] -> w252
          tunnel: w250 -> [w273 w288]
          tunnel: w249 -> [w280 w290]
          tunnel: w248 -> [w279 w289]
          tunnel: w247 -> [w278 _]
          tunnel: w246 -> [w277 _]
          tunnel: w245 -> [w275 _]
          tunnel: [w273 w288] -> w244
          tunnel: w243 -> [w272 w287]
          tunnel: w242 -> [_ w286]
          tunnel: w241 -> [_ w285]
          tunnel: [w272 w283] -> w240
          tunnel: w239 -> [_ w282]
          frame "T2", Default {
          }
          frame "Rabi" {
            n141 = Bundle By Name(cluster=w288, "MW_width_us"=w302, "pulse_width_us"=w307, "read_delay_us"=w308, "read_width_us"=w306, "repetitions"=w305, "sampling_mode"=w304, "correction_us"=w303) -> (w300:T3)
            n142 = Bundle By Name(cluster=w287, "MW_power_db"=w286, "MW_frequency_GHZ"=w285) -> (w283:T2)
            n143 = property on="elapsed_time_HMS" class="Str"("Value"="") -> (error out=w298:errorcluster)  [unwired: 2 in, 1 out]
            n144 = flat-sequence {
              tunnel: w300 -> [w317]
              tunnel: [w317] -> w313
              tunnel: [w316] -> w312
              tunnel: w298 -> [_]
              tunnel: w283 -> [w315]
              tunnel: [w315] -> w284
              tunnel: w282 -> [w314]
              tunnel: [w314] -> w281
              tunnel: [w322] -> w309
              tunnel: [w321] -> w299
              tunnel: w313 -> [w324]
              tunnel: [w320] -> w311
              tunnel: [w325] -> w310
              tunnel: w312 -> [w325]
              tunnel: w295 -> [w323]
              tunnel: w284 -> [w319]
              tunnel: w281 -> [w318]
              tunnel: [w329] -> w301
              tunnel: w311 -> [w329]
              tunnel: w310 -> [w327]
              tunnel: [w326] -> w296
              frame #0 {
                n145 = Tick Count (ms)() -> (millisecond timer value=w316:u32)
              }
              frame #1 {
                n146 = call "doRabi.vi"("q_samples"=w318, "MW_Parameters"=w319, "parameters_recenter"=w323, "Rabi_parameters"=w324) -> ("triggers"=w321:u32[][], "Rabi_curve"=w320:cluster{dbl[], "dark_time_us":dbl[]}, "timetags"=w322:u32[][])  [unwired: 4 in, 1 out]
              }
              frame #2 {
                n147 = Tick Count (ms)() -> (millisecond timer value=w328:u32)
                n148 = Subtract(x=w328, y=w327) -> (x-y=w326:u32)
              }
            }
            n149 = Bundle By Name(cluster=T9 {"input_xyz"={"nano-position_X_um"=0.0, "nano-position_Y_um"=0.0, "nano-position Z_um"=0.0}, "recenter"=FALSE, "recenter_s"=3} ("parameters_recenter"), "input_xyz"="input_xyz", "recenter"="recenter", "recenter_s"="recenter_period_s") -> (w295:T9)
          }
        }
        n150 = Multiply(x=w254, y=0.001) -> (x*y=w259:dbl)
        n151 = call "seconds2time.vi"("seconds"=w259) -> ("HH:MM:SS"=w255:string)  [unwired: 10 in]
        "elapsed_time_HMS" <- w255
        n152 = flat-sequence {
          tunnel: w255 -> [_]
          frame #0 {
            n153 = property on="status" class="Str"("Value"="") -> ()  [unwired: 2 in, 2 out]
            n154 = call "laserON-OFF.vi"("ON-OFF"=TRUE) -> ()  [unwired: 11 in]
          }
        }
      }
      frame "abort" {
      }
      frame "calcWidth" {
        n155 = call "find_read_width.vi"("timetags"=w352, "T1_parameters"=w351) -> ("mse"=→"mse":cluster{"read_widths_us":dbl[], "mse":dbl[]}, "proposed_read_width_us"=w347:dbl)  [unwired: 8 in]
        "proposed_read_width_us" <- w347
        n156 = flat-sequence {
          tunnel: w347 -> [_]
          frame #0 {
            n157 = property on="status" class="Str"("Value"="") -> ()  [unwired: 2 in, 2 out]
          }
        }
      }
    }
  }
